vi "Test SendLogRecordsDoesNotThrowError.vi"(8 "error in (no error)":errorcluster) -> (0 "error out":errorcluster)   [LabVIEW 2017, in "UT_LokiHandler.lvlib"]
doc: "Template for an unit test with caraya in the \"Given, When, Then\" structure from James."
uses:
  UT_LokiHandler.lvlib
  Source/HSE-Logger/Handler/LokiHandler/LokiHandler.lvclass
  <vilib>/addons/_JKI Toolkits/Caraya/classes/Test/Test.lvclass
  <vilib>/addons/_JKI Toolkits/Caraya/classes/Assert/Assert.lvclass
  <vilib>/addons/_JKI Toolkits/Caraya/classes/Assert/Assert Not Error.vi
  Source/HSE-Logger/LogRecord/LogRecord.lvclass
  Source/HSE-Logger/LogLevel.ctl
  Source/HSE-Logger/hse-logger.lvlib
panel:
  # "Connector Pane"
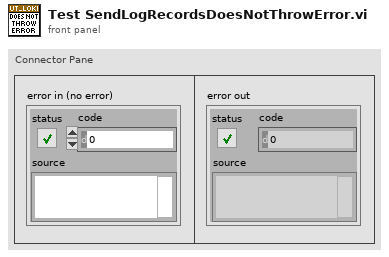
[diagram p1: front panel]
types:
  T1 = typedef "hse-logger.lvlib/LogLevel.ctl" = enum16{"DEBUG", "INFO", "WARNING", "ERROR", "CRITICAL"}
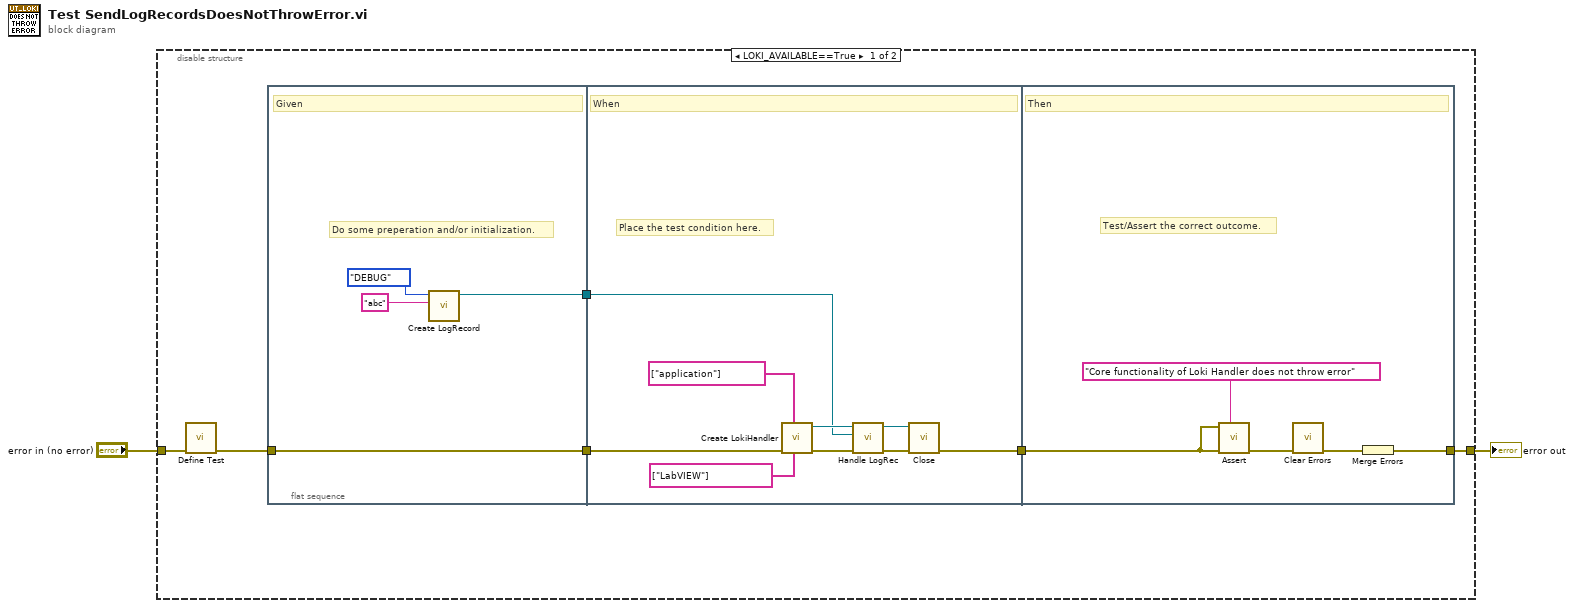
[diagram p0: block diagram]
diagram:
  n1 = disable-structure shown="LOKI_AVAILABLE==True" {
    disable-tunnel: [w6 w27] -> w2
    disable-tunnel: "error in (no error)" -> [w5 w27]
    frame condition #0 (active) {
      n2 = call <vilib>:"Define Test.vi"("error in (no error)"=w5) -> ("error out"=w4:errorcluster)  [unwired: 9 in, 1 out]
      n3 = flat-sequence {
        tunnel: w4 -> [w12]
        tunnel: [w12] -> w8
        tunnel: [w9] -> w3
        tunnel: w8 -> [w17]
        tunnel: [w16] -> w7
        tunnel: w3 -> [w13]
        tunnel: [w25] -> w6
        tunnel: w7 -> [w23]
        frame #0 {
          # "Do some preperation and/or initialization."
          # "Given"
          n4 = call "Create LogRecord.vi"("Message"="abc", "Level"=LogLevel."DEBUG") -> ("LogRecord out"=w9:refnum<class "LogRecord.lvclass">)  [unwired: 8 in, 1 out]
        }
        frame #1 {
          # "Place the test condition here."
          # "When"
          n5 = call "Create LokiHandler.vi"("Stream Fields Values"=string[] ["LabVIEW"], "Stream Fields"=string[] ["application"], "error in"=w17) -> ("error out"=w19:errorcluster, "LokiHandler out"=w18:refnum<class "LokiHandler.lvclass">)  [unwired: 7 in]
          n6 = call-dynamic "Handle LogRec.vi"("error in"=w19, "LogRecord"=w13, "LokiHandler in"=w18) -> ("error out"=w15:errorcluster, "LokiHandler out"=w14:refnum<class "LokiHandler.lvclass">)  [unwired: 7 in]
          n7 = call-dynamic "Close.vi"("error in"=w15, "LokiHandler in"=w14) -> ("error out"=w16:errorcluster)  [unwired: 8 in, 1 out]
        }
        frame #2 {
          # "Test/Assert the correct outcome."
          # "Then"
          n8 = call-poly <vilib>:"Assert.vi"("Label"="Core functionality of Loki Handler does not throw error", "error in (no error)"=w23, "Not Error?"=w23) -> ("error out"=w26:errorcluster)  [unwired: 7 in, 1 out]
          n9 = call <vilib>:"Clear Errors.vi"("error in (no error)"=w26) -> ("error out"=w22:errorcluster)  [unwired: 5 in, 1 out]
          n10 = Merge Errors(w22) -> (w25:errorcluster)
        }
      }
    }
    frame condition #1 {
    }
  }
  "error out" <- w2
